vi "setCamera.vi"(8 "error in (no error)":errorcluster, 10 "Camera":refnum<class "Camera.lvclass">, 11 "NetworkCamera in":refnum<class "NetworkCamera.lvclass">) -> (0 "error out":errorcluster, 3 "NetworkCamera out":refnum<class "NetworkCamera.lvclass">)   [LabVIEW 2011, in "Hardware.lvlib" / "HWControllers.lvlib" / "NetworkCamera.lvclass"]
uses:
  NetworkCamera.lvclass
  Channels/Camera/Camera/Camera.lvclass
  NetworkCamera.lvclass/NetworkCamera.ctl
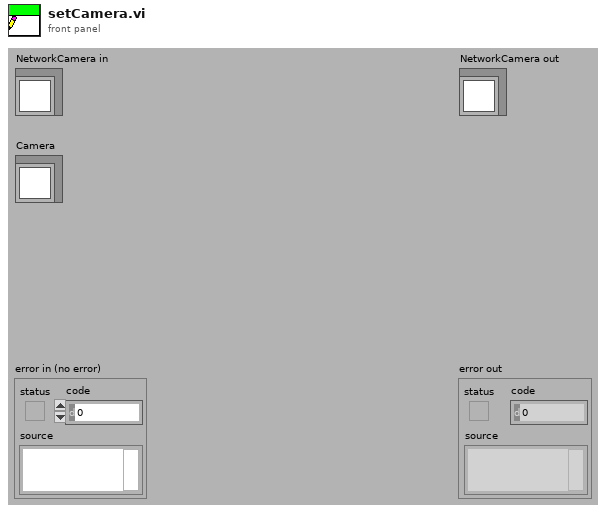
[diagram p1: front panel]
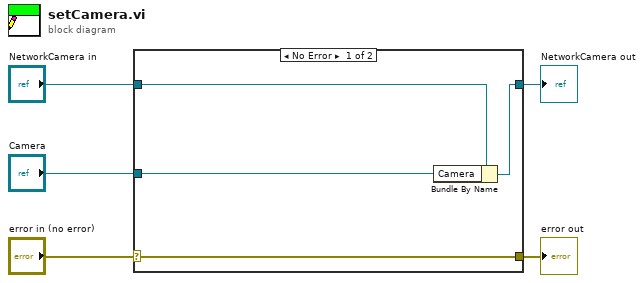
[diagram p0: block diagram]
diagram:
  n1 = case shown="No Error" "error in (no error)" {
    selector: "error in (no error)" -> [w9 w10]
    tunnel: [w9 w10] -> w4
    tunnel: [w7 w11] -> w2
    tunnel: "NetworkCamera in" -> [w8 w11]
    tunnel: "Camera" -> [w6 _]
    frame No Error {
      n2 = Bundle By Name(cluster=w8, "Camera"=w6) -> (w7:refnum<class "NetworkCamera.lvclass">)
    }
    frame Error {
    }
  }
  "error out" <- w4
  "NetworkCamera out" <- w2
